vi "addSkipped.vi"(8 "error in (no error)":errorcluster, 10 "test":refnum<class>, 11 "TestTestResult in":refnum<class "_TextTestResult.JUnitXML.lvclass">) -> (0 "error out":errorcluster, 3 "TestTestResult out":refnum<class "_TextTestResult.JUnitXML.lvclass">)   [LabVIEW 2011, in "_TextTestResult.JUnitXML.lvclass"]
uses:
  _TextTestResult.JUnitXML.lvclass
  <vilib>/addons/_JKI Toolkits/VI Tester/TestResult.llb/resultStatus--enum.ctl
  <vilib>/addons/_JKI Toolkits/VI Tester/_TextTestResult.llb/_TextTestResult.lvclass
  <vilib>/addons/_JKI Toolkits/VI Tester/TestResult.llb/TestResult.lvclass
panel:
  # "JKI VI Tester for LabVIEW\nhttp://jkisoft.com/vi-tester\nCopyright (C) 2007-2009, JKI <info@jkisoft.com>\nALL RIGHTS RESERVED"
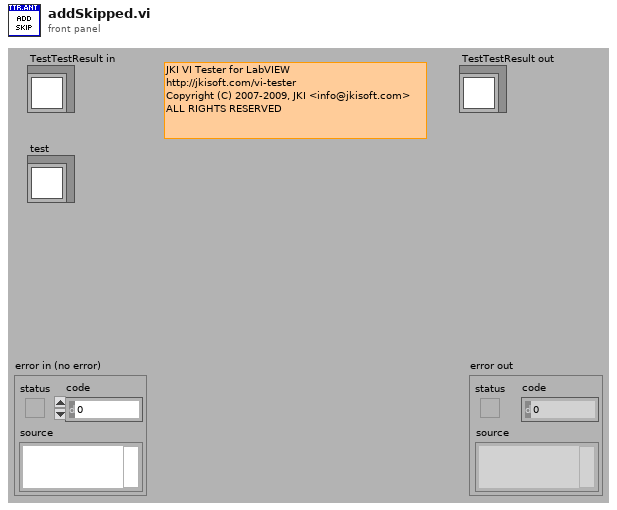
[diagram p1: front panel]
types:
  T1 = typedef "TestResult.lvclass/resultStatus--enum.ctl" = enum16{"testPass", "testFailure", "testError", "testSkipped"}
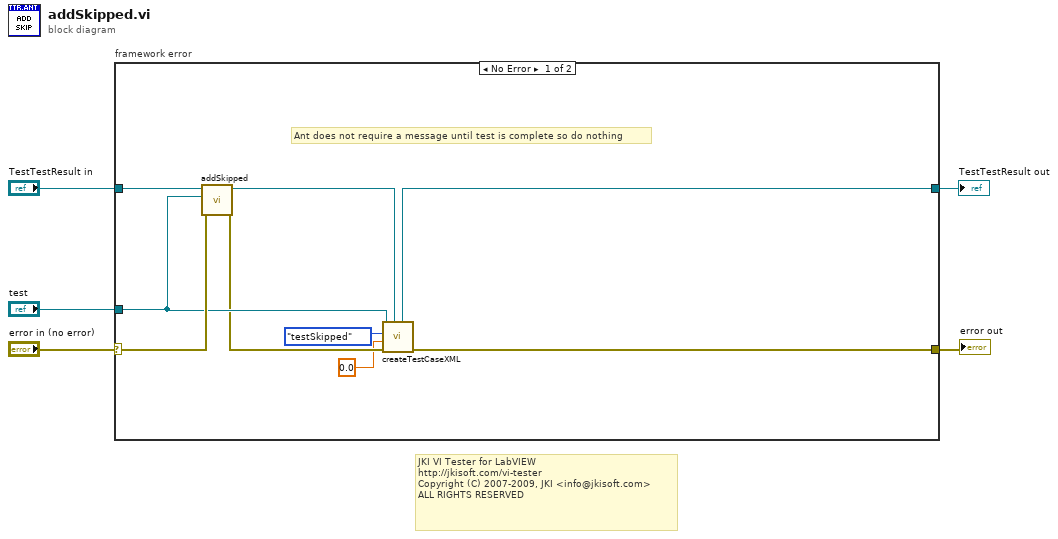
[diagram p0: block diagram]
diagram:
  # "JKI VI Tester for LabVIEW\nhttp://jkisoft.com/vi-tester\nCopyright (C) 2007-2009, JKI <info@jkisoft.com>\nALL RIGHTS RESERVED"
  n1 = case "framework error" shown="No Error" "error in (no error)" {
    selector: "error in (no error)" -> [w13 w16]
    tunnel: [w8 w16] -> w4
    tunnel: [w6 w15] -> w2
    tunnel: "TestTestResult in" -> [w14 w15]
    tunnel: "test" -> [w11 _]
    frame No Error {
      # "Ant does not require a message until test is complete so do nothing"
      n2 = call-parent "addSkipped.vi"("error in (no error)"=w13, "test"=w11, "TestTestResult in"=w14) -> ("error out"=w10:errorcluster, "TestTestResult out"=w7:refnum<class "_TextTestResult.JUnitXML.lvclass">)  [unwired: 7 in]
      n3 = call "createTestCaseXML.vi"("TestTestResult.Ant"=w7, "error in (no error)"=w10, "execution time (sec)"=0.0, "resultStatus"=resultStatus--enum."testSkipped", "Test Out"=w11) -> ("error out"=w8:errorcluster, "TestTestResult.Ant Out"=w6:refnum<class "_TextTestResult.JUnitXML.lvclass">)  [unwired: 5 in]
    }
    frame Error {
    }
  }
  "error out" <- w4
  "TestTestResult out" <- w2
